vi "Read AItasks# 2.vi"(8 "error in (no error)":errorcluster, 11 "DAQmxTaksContainer_General in":refnum<class "DAQmxTaksContainer_General.lvclass">) -> (0 "error out":errorcluster, 2 "AItasks#":i32, 3 "DAQmxTaksContainer_General out":refnum<class "DAQmxTaksContainer_General.lvclass">)   [LabVIEW 2015]
uses:
  DAQmxTaksContainer_General.lvclass
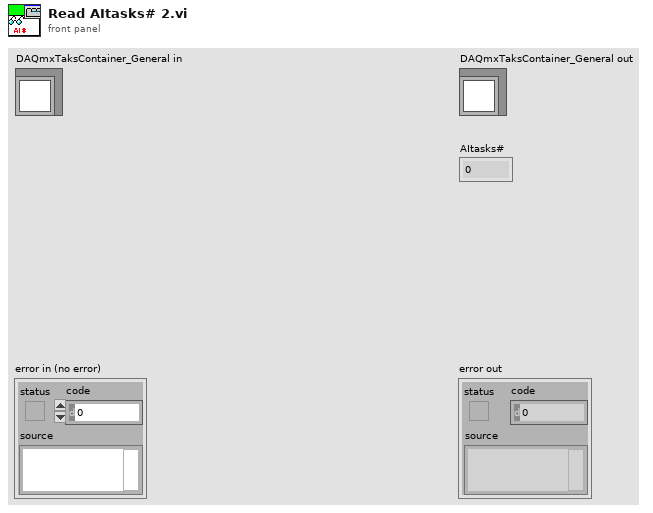
[diagram p1: front panel]
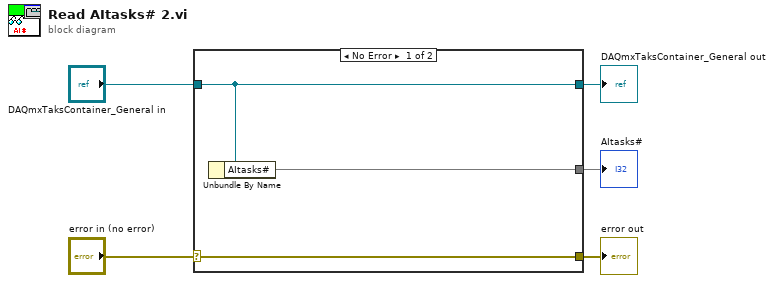
[diagram p0: block diagram]
diagram:
  n1 = case shown="No Error" "error in (no error)" {
    selector: "error in (no error)" -> [w8 w9]
    tunnel: [w8 w9] -> w4
    tunnel: [w7 w10] -> w2
    tunnel: "DAQmxTaksContainer_General in" -> [w7 w10]
    tunnel: [w6 _] -> w1
    frame No Error {
      n2 = Unbundle By Name(w7) -> ("AItasks#"=w6)
    }
    frame Error {
    }
  }
  "error out" <- w4
  "DAQmxTaksContainer_General out" <- w2
  "AItasks#" <- w1
